vi "SETMIXdll.vi"(8 "error in (no error)":errorcluster, 11 "Inputs":T2) -> (0 "error out":errorcluster, 3 "Outputs":T1)   [LabVIEW 2015]
doc: "subroutine SETMIXdll(hmxnme, hfmix, hrf, ncc, hfile, z, ierr, herr, hmxnme_length, hfmix_length,\nhrf_length, hfile_length, herr_length)\n\nOpen a mixture file (e.g., R410A.mix) and read constituents and mole fractions.\n\nINPUTS:\nhmxnme -- Mixture file name (character*255)\nhfmix -- File containing mixture coefficients (character*255)\nhrf -- Reference state (character*3) (see subroutine SETUP for specifics)\n\nOUTPUTS:\nncc -- Number of fluids in mixture\nhfile -- array of file names specifying mixture components that were used to call setup.\nz -- Array of mole fractions for the specified mixture\nierr -- Error flag: 0 - Successful \n 101 - Error in opening file \n -102 - Mixture file contains mixing parameters \n -104 - Sum of compositions not equal to one\nherr -- Error string (character*255)\nhmxnme_length -- length of variable hmxnme (default: 255)\nhfmix_length -- length of variable hfmix (default: 255)\nhrf_length -- length of variable hrf (default: 3)\nhfile_length -- length of variable hfile (default: 10000)\nherr_length --length of variable herr (default: 255)"
uses:
  REFPROP.dll
panel:
  # "REFPROP-SETMIXdll.vi"
  # "void  SETMIXdll(CStr hmxnme, CStr hfmix, CStr hrf, int32_t *ncc, CStr hfile, double *z, int32_t *ierr, CStr herr, int32_t hmxnme_length, int32_t hfmix_length, int32_t hrf_length, int32_t hfile_length, int32_t herr_length)"
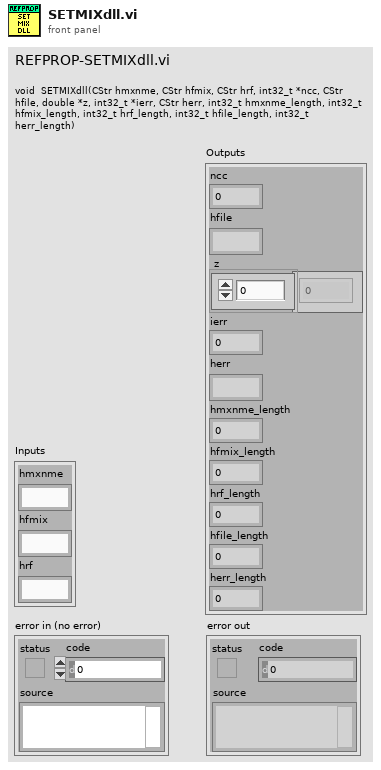
[diagram p1: front panel]
types:
  T1 = cluster{"ncc":i32, "hfile":string, "z":dbl[], "ierr":i32, "herr":string, "hmxnme_length":i32, "hfmix_length":i32, "hrf_length":i32, "hfile_length":i32, "herr_length":i32}
  T2 = cluster{"hmxnme":string, "hfmix":string, "hrf":string}
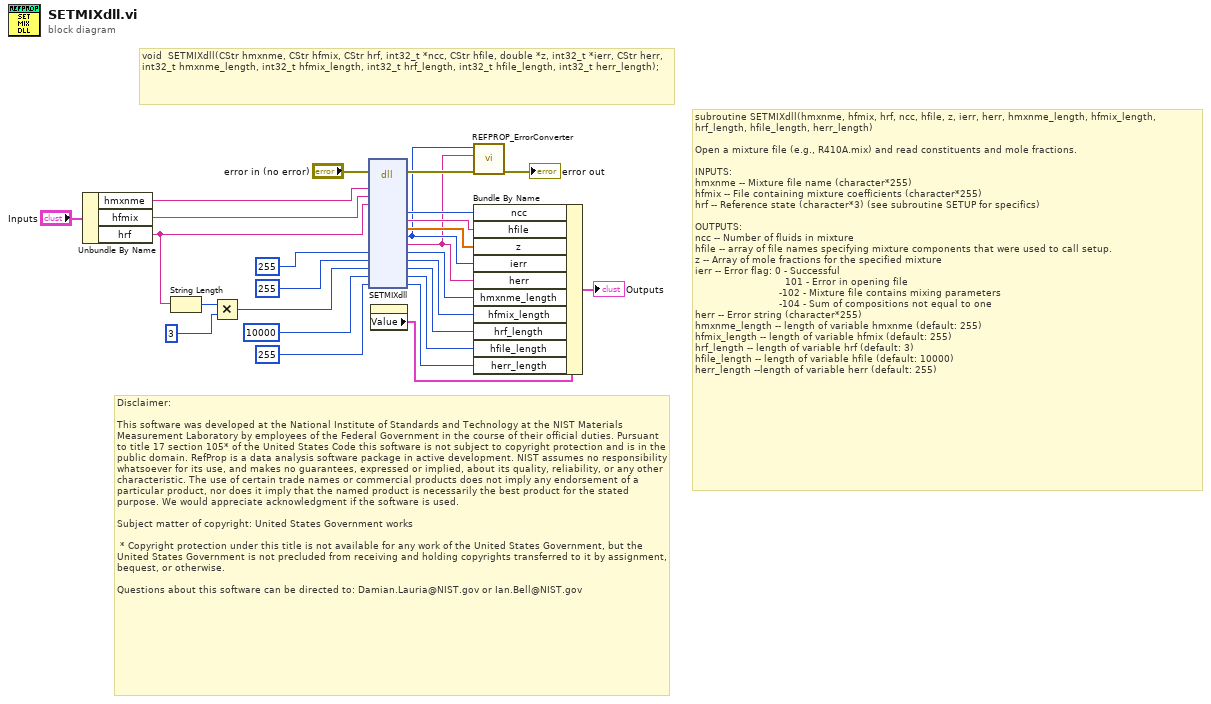
[diagram p0: block diagram]
diagram:
  # "Disclaimer:\n\nThis software was developed at the National Institute of Standards and Technology at the NIST Materials Measurement Laboratory by employees of the Federal Government in the course of their official duties. Pursuant to title 17 section 105* of the United States Code this software is not subject to copyright protection and is in the public domain. RefProp is a data analysis software package in active development. NIST assumes no responsibility whatsoever for its use, and makes no guarantees, expressed or implied, about its quality, reliability, or any other characteristic. The use of certain trade names or commercial products does not imply any endorsement of a particular product, nor does it imply that the named product is necessarily the best product for the stated purpose. We would appreciate acknowledgment if the software is used.\n \nSubject matter of copyright: United States Government works\n  \n * Copyright protection under this title is not available for any work of the United States Government, but the United States Government is not precluded from receiving and holding copyrights transferred to it by assignment, bequest, or otherwise.\n\nQuestions about this software can be directed to: Damian.Lauria@NIST.gov or Ian.Bell@NIST.gov"
  # "void  SETMIXdll(CStr hmxnme, CStr hfmix, CStr hrf, int32_t *ncc, CStr hfile, double *z, int32_t *ierr, CStr herr, int32_t hmxnme_length, int32_t hfmix_length, int32_t hrf_length, int32_t hfile_length, int32_t herr_length);"
  # "subroutine SETMIXdll(hmxnme, hfmix, hrf, ncc, hfile, z, ierr, herr, hmxnme_length, hfmix_length,\nhrf_length, hfile_length, herr_length)\n\nOpen a mixture file (e.g., R410A.mix) and read constituents and mole fractions.\n\nINPUTS:\nhmxnme -- Mixture file name (character*255)\nhfmix -- File containing mixture coefficients (character*255)\nhrf -- Reference state (character*3) (see subroutine SETUP for specifics)\n\nOUTPUTS:\nncc -- Number of fluids in mixture\nhfile -- array of file names specifying mixture components that were used to call setup.\nz -- Array of mole fractions for the specified mixture\nierr -- Error flag: 0 - Successful \n                              101 - Error in opening file \n                            -102 - Mixture file contains mixing parameters \n                            -104 - Sum of compositions not equal to one\nherr -- Error string (character*255)\nhmxnme_length -- length of variable hmxnme (default: 255)\nhfmix_length -- length of variable hfmix (default: 255)\nhrf_length -- length of variable hrf (default: 3)\nhfile_length -- length of variable hfile (default: 10000)\nherr_length --length of variable herr (default: 255)"
  n1 = Unbundle By Name("Inputs") -> ("hmxnme"=w22:string, "hfmix"=w21:string, "hrf"=w3:string)
  n2 = String Length(string=w3) -> (length=w4:i32)
  n3 = Multiply(x=w4, y=3) -> (x*y=w1:i32)
  n4 = dll-call lib="C:/Users/lauria/Desktop/REFPROP 10 LabVIEW Wrapper BETA/REFPROP/REFPROP.*" fn="SETMIXdll"(error in="error in (no error)", "hmxnme"=w22, "hfmix"=w21, "hrf"=w3, "hmxnme_length"=255, "hfmix_length"=255, "hrf_length"=w1, "hfile_length"=10000, "herr_length"=255) -> (error out=w26:errorcluster, "ncc"=w18:i32, "hfile"=w17:string, "z"=w16:dbl[], "ierr"=w10:i32, "herr"=w9:string, "hmxnme_length"=w15:i32, "hfmix_length"=w14:i32, "hrf_length"=w13:i32, "hfile_length"=w12:i32, "herr_length"=w11:i32)  [unwired: 11 in, 1 out]
  n5 = property on="Outputs" class="Clust (strict)"() -> ("Value"=w19:T1)  [unwired: 2 in, 2 out]
  n6 = call "REFPROP_ErrorConverter.vi"("error in (no error)"=w26, "Error Message"=w9, "Error Code"=w10) -> ("error out"=→"error out":errorcluster)  [unwired: 8 in]
  n7 = Bundle By Name(cluster=w19, "ncc"=w18, "hfile"=w17, "z"=w16, "ierr"=w10, "herr"=w9, "hmxnme_length"=w15, "hfmix_length"=w14, "hrf_length"=w13, "hfile_length"=w12, "herr_length"=w11) -> (→"Outputs":T1)
